vi "generate galvo waveforms.vi"(8 "error in (no error)":errorcluster, 11 "Waveform in":refnum<class "Waveform.lvclass">) -> (0 "error out":errorcluster, 1 "Waveform 2":waveform(dbl), 2 "Waveform":waveform(dbl), 3 "Waveform out":refnum<class "Waveform.lvclass">)   [LabVIEW 2012, in "Waveform.lvclass"]
uses:
  Waveform.lvclass
  Waveform.lvclass/Waveform.ctl
panel:
  out "wfm2":waveform(dbl)(graph)
  out "wfm1":waveform(dbl)(graph)
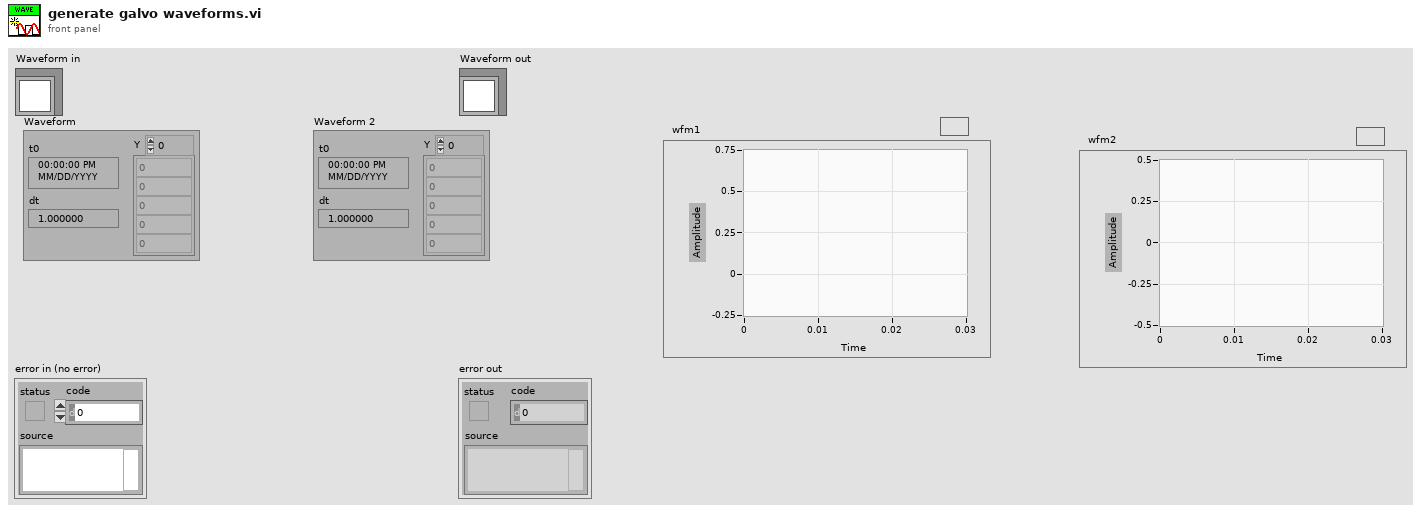
[diagram p1: front panel]
types:
  T1 = typedef "Waveform.lvclass/waveform data.ctl" = cluster{"amplitude":dbl[unit], "offset":dbl[unit], "delay":dbl[unit], "duty cycle":dbl, "sampling info":cluster{"Fs":dbl, "#s":dbl}, "frequency":dbl[unit], "phase":dbl[unit]}
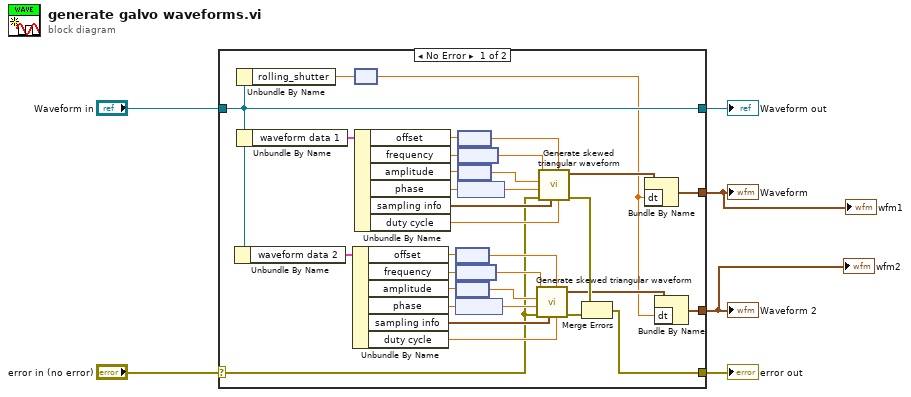
[diagram p0: block diagram]
diagram:
  n1 = case shown="No Error" "error in (no error)" {
    selector: "error in (no error)" -> [w17 w41]
    tunnel: [w16 w41] -> w5
    tunnel: [w15 w40] -> w3
    tunnel: "Waveform in" -> [w15 w40]
    tunnel: [w10 _] -> w2
    tunnel: [w9 _] -> w1
    frame No Error {
      n2 = Unbundle By Name(w15) -> ("waveform data 2"=w22:T1)
      n3 = Unbundle By Name(w15) -> ("rolling_shutter"=w14:dbl[unit])
      n4 = Unbundle By Name(w15) -> ("waveform data 1"=w39:T1)
      n5 = Unbundle By Name(w22) -> ("offset"=w24:dbl[unit], "frequency"=w25:dbl[unit], "amplitude"=w7:dbl[unit], "phase"=w28:dbl[unit], "sampling info"=w30:cluster{"Fs":dbl, "#s":dbl}, "duty cycle"=w20:dbl)
      n6 = node(w14) -> (w11:dbl)
      n7 = Unbundle By Name(w39) -> ("offset"=w37:dbl[unit], "frequency"=w36:dbl[unit], "amplitude"=w8:dbl[unit], "phase"=w33:dbl[unit], "sampling info"=w31:cluster{"Fs":dbl, "#s":dbl}, "duty cycle"=w21:dbl)
      n8 = node(w24) -> (w23:dbl)
      n9 = node(w25) -> (w26:dbl)
      n10 = node(w7) -> (w27:dbl)
      n11 = node(w28) -> (w29:dbl)
      n12 = node(w37) -> (w38:dbl)
      n13 = node(w36) -> (w35:dbl)
      n14 = node(w8) -> (w34:dbl)
      n15 = node(w33) -> (w32:dbl)
      n16 = call "Generate skewed triangular waveform.vi"("Duty cycle (%)"=w20, "Offset"=w23, "sampling info"=w30, "error in (no error)"=w17, "Phase"=w29, "Amplitude"=w27, "Frequency"=w26) -> ("error out"=w18:errorcluster, "Waveform"=w12:waveform(dbl))  [unwired: 3 in]
      n17 = call "Generate skewed triangular waveform.vi"("Duty cycle (%)"=w21, "Offset"=w38, "sampling info"=w31, "error in (no error)"=w17, "Phase"=w32, "Amplitude"=w34, "Frequency"=w35) -> ("error out"=w19:errorcluster, "Waveform"=w13:waveform(dbl))  [unwired: 3 in]
      n18 = Merge Errors(w19, w18) -> (w16:errorcluster)
      n19 = Bundle By Name(cluster=w13, "dt"=w11) -> (w10:waveform(dbl))
      n20 = Bundle By Name(cluster=w12, "dt"=w11) -> (w9:waveform(dbl))
    }
    frame Error {
    }
  }
  "error out" <- w5
  "Waveform out" <- w3
  "Waveform" <- w2
  "Waveform 2" <- w1
  "wfm1" <- w2
  "wfm2" <- w1
